vi "Test Gain.vi"(8 "error in (no error)":errorcluster, 11 "Instrument.Lockin in":refnum<class "Instrument.Lockin.lvclass">) -> (0 "error out":errorcluster, 3 "Instrument.Lockin out":refnum<class "Instrument.Lockin.lvclass">)   [LabVIEW 2019]
uses:
  src/Instrument.Lockin/Instrument.Lockin.lvclass
  <vilib>/addons/_JKI Toolkits/Caraya/classes/Assert/Assert Equal Value_Variant.vi
  <vilib>/addons/_JKI Toolkits/Caraya/classes/Test/Test.lvclass
  <vilib>/addons/_JKI Toolkits/Caraya/classes/Assert/Assert.lvclass
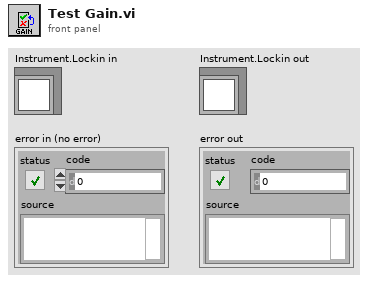
[diagram p1: front panel]
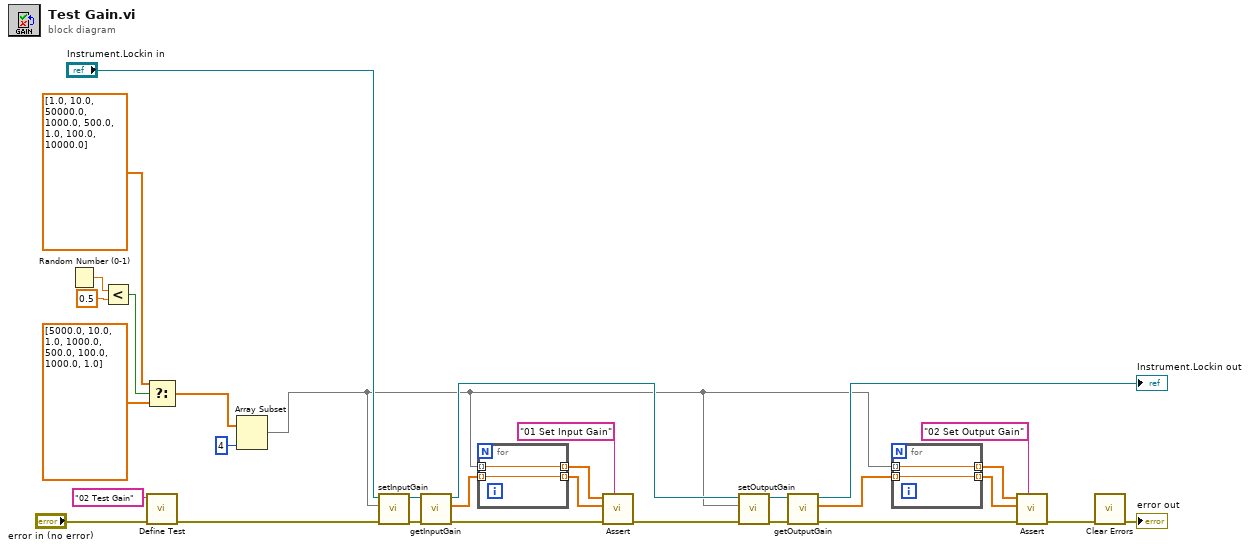
[diagram p0: block diagram]
diagram:
  n1 = Random Number (0-1)() -> (number: 0 to 1=w26:dbl)
  n2 = Less?(x=w26, y=0.5) -> (x < y?=w23:bool)
  n3 = Select(t=dbl[] [1.0, 10.0, 50000.0, 1000.0, 500.0, 1.0, 100.0, 10000.0] ("Gain"), s=w23, f=dbl[] [5000.0, 10.0, 1.0, 1000.0, 500.0, 100.0, 1000.0, 1.0] ("Gain")) -> (s? t:f=w3:dbl[])
  n4 = call <vilib>:"Define Test.vi"("error in (no error)"="error in (no error)", "Label (VI Title)"="02 Test Gain") -> ("error out"=w31:errorcluster)  [unwired: 8 in, 1 out]
  n5 = Array Subset(array=w3, length=4) -> (w2:dbl[])  [unwired: 1 in]
  n6 = call-dynamic "setInputGain.vi"("error in (no error)"=w31, "InputGain"=w2, "Instrument.Lockin in"="Instrument.Lockin in") -> ("error out"=w29:errorcluster, "Instrument.Lockin out"=w28:refnum<class "Instrument.Lockin.lvclass">)  [unwired: 7 in]
  n7 = call-dynamic "getInputGain.vi"("error in (no error)"=w29, "Instrument.Lockin in"=w28) -> ("error out"=w16:errorcluster, "InputGain"=w19:dbl[], "Instrument.Lockin out"=w12:refnum<class "Instrument.Lockin.lvclass">)  [unwired: 7 in]
  n8 = for {
    tunnel: [w33] -> w18 mode=indexing
    tunnel: w2 -> [w33] mode=indexing
    tunnel: [w32] -> w17 mode=indexing
    tunnel: w19 -> [w32] mode=indexing
  }
  n9 = call-poly <vilib>:"Assert.vi"("Label"="01 Set Input Gain", "error in (no error)"=w16, "Actual"=w17, "Expected"=w18) -> ("error out"=w14:errorcluster)  [unwired: 6 in, 1 out]
  n10 = call-dynamic "setOutputGain.vi"("error in (no error)"=w14, "OutputGain"=w2, "Instrument.Lockin in"=w12) -> ("error out"=w13:errorcluster, "Instrument.Lockin out"=w6:refnum<class "Instrument.Lockin.lvclass">)  [unwired: 7 in]
  n11 = call-dynamic "getOutputGain.vi"("error in (no error)"=w13, "Instrument.Lockin in"=w6) -> ("error out"=w8:errorcluster, "OutputGain"=w7:dbl[], "Instrument.Lockin out"=→"Instrument.Lockin out":refnum<class "Instrument.Lockin.lvclass">)  [unwired: 7 in]
  n12 = for {
    tunnel: [w35] -> w9 mode=indexing
    tunnel: w2 -> [w35] mode=indexing
    tunnel: [w34] -> w10 mode=indexing
    tunnel: w7 -> [w34] mode=indexing
  }
  n13 = call-poly <vilib>:"Assert.vi"("Label"="02 Set Output Gain", "error in (no error)"=w8, "Actual"=w10, "Expected"=w9) -> ("error out"=w4:errorcluster)  [unwired: 6 in, 1 out]
  n14 = call <vilib>:"Clear Errors.vi"("error in (no error)"=w4) -> ("error out"=→"error out":errorcluster)  [unwired: 5 in, 1 out]
